vi "Boolean Assert Test.vi"(11 "Data In":bool) -> (3 "Data Out":bool)   [LabVIEW 2016]
uses:
  Core/Assert API Components/Failure Actions.ctl
  Core/Assert API Components/Assert API Components.lvlib
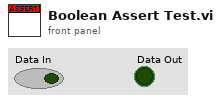
[diagram p1: front panel]
types:
  T1 = typedef "Assert API Components.lvlib/Failure Actions.ctl" = enum16{"None", "Log To File", "Pause Execution", "Abort Execution"}
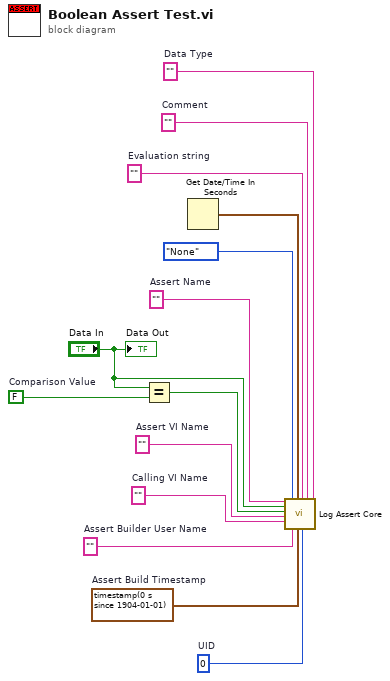
[diagram p0: block diagram]
diagram:
  w1 = 0  # UID
  w4 = ""  # Assert VI Name
  w5 = ""  # Calling VI Name
  w6 = timestamp(0 s since 1904-01-01)  # Assert Build Timestamp
  w7 = ""  # Assert Builder User Name
  w8 = ""  # Data Type
  w13 = ""  # Comment
  w12 = ""  # Evaluation string
  w14 = ""  # Assert Name
  w10 = FALSE  # Comparison Value
  n1 = Equal?(x="Data In", y=w10) -> (x = y?=w9:bool)
  n2 = Get Date/Time In Seconds() -> (seconds since 1Jan1904=w2:timestamp)
  n3 = call "Log Assert Core.vi"("Assert Name"=w14, "Data Value"="Data In", "Status"=w9, "Assert VI Name"=w4, "Calling VI Name"=w5, "Failure Action"=Failure_Actions."None" ("Default Failure Action"), "Assert Builder User Name"=w7, "Last Update"=w2, "Assert Build Timestamp"=w6, "Evaluation String"=w12, "Assert VI UID"=w1, "Comment"=w13, "Data Type"=w8) -> ()  [unwired: 7 in]
  "Data Out" <- "Data In"
